vi "Timed Message.vi"(9 "Interval (ms)":u32, 10 "State":string, 11 "Queue in":refnum<queue>) -> ()   [LabVIEW 2026]
uses:
  Type Defs/Queue Data.ctl
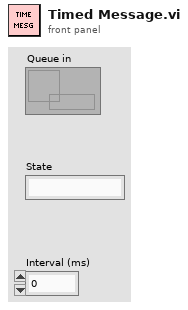
[diagram p1: front panel]
types:
  T1 = typedef "Queue Data.ctl" = cluster{"State":string, "Data":variant}
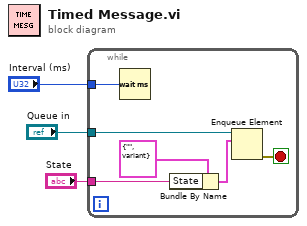
[diagram p0: block diagram]
diagram:
  n1 = while {
    tunnel: "Queue in" -> [w7]
    tunnel: "Interval (ms)" -> [w5]
    tunnel: "State" -> [w4]
    stop <- w6 stop-if-true
    n2 = Wait (ms)(milliseconds to wait=w5) -> ()  [unwired: 1 out]
    n3 = Bundle By Name(cluster=T1 {"State"="", "Data"=variant} ("element"), "State"=w4) -> (w9:T1)
    n4 = Enqueue Element(queue=w7, element=w9) -> (error out=w6:errorcluster)  [unwired: 2 in, 2 out]
  }
